vi "Write X-t Value Pairs.vi"(8 "Error In":errorcluster, 10 "X-t Value Pairs":cluster{"Time Stamp":timestamp, "Value":dbl}[](array[cluster]) {"Time Stamp" format="%<%x %.3X>T"}, 11 "Add Timestamped Data Msg":refnum<class "Add Timestamped Data Msg.lvclass">) -> (0 "Error Out":errorcluster, 3 "Add Timestamped Data Msg":refnum<class "Add Timestamped Data Msg.lvclass">)   [LabVIEW 2018, in "BNT_XtGraph.lvlib" / "Add Timestamped Data Msg.lvclass"]
uses:
  Add Timestamped Data Msg.lvclass
  Add Timestamped Data Msg.lvclass/Add Timestamped Data Msg.ctl
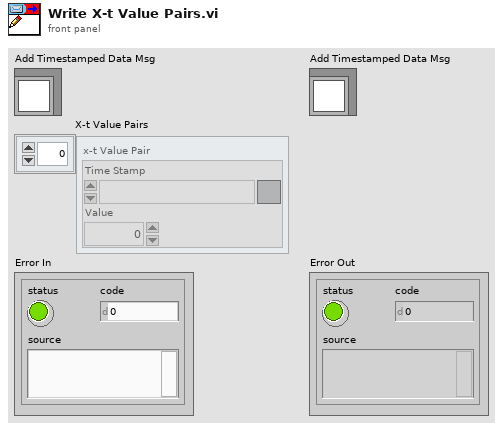
[diagram p1: front panel]
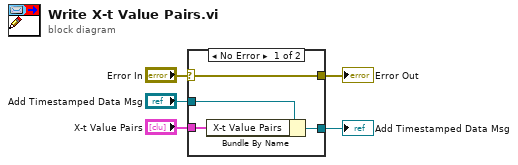
[diagram p0: block diagram]
diagram:
  n1 = case shown="No Error" "Error In" {
    selector: "Error In" -> [w9 w10]
    tunnel: [w9 w10] -> w5
    tunnel: [w7 w11] -> w3
    tunnel: "Add Timestamped Data Msg" -> [w8 w11]
    tunnel: "X-t Value Pairs" -> [w6 _]
    frame No Error {
      n2 = Bundle By Name(cluster=w8, "X-t Value Pairs"=w6) -> (w7:refnum<class "Add Timestamped Data Msg.lvclass">)
    }
    frame Error {
    }
  }
  "Add Timestamped Data Msg" <- w3
  "Error Out" <- w5
